vi "PathPlanner_CurrentTrigEventMarkers_FGV.vi"(10 "in EventMarkers":T1[](array[typedef]) {"lastRobotPos"."Y" format="%14.3f"; "lastRobotPos"."X" format="%14.3f"; "markerPos"."Y" format="%14.3f"; "markerPos"."X" format="%14.3f"}, 11 "Write":bool) -> (2 "out EventMarkers":T1[](array[typedef]) {"lastRobotPos"."Y" format="%14.3f"; "lastRobotPos"."X" format="%14.3f"; "markerPos"."Y" format="%14.3f"; "markerPos"."X" format="%14.3f"})   [LabVIEW 2023]
uses:
  <vilib>/Rock Robotics/WPI/ThirdParty/JAS_Junk/TrajLib/TypeDef/TRANSLATION2D.ctl
  <vilib>/Rock Robotics/WPI/ThirdParty/JAS_Junk/TrajLib/Trajectory_Library.lvlib
  <vilib>/Rock Robotics/WPI/ThirdParty/MJansen/PathPlanner/ENum/PathPlanner_CommandUtilType_ENUM.ctl
  <vilib>/Rock Robotics/WPI/ThirdParty/MJansen/PathPlanner/PathPlanner24.lvlib
  <vilib>/Rock Robotics/WPI/ThirdParty/MJansen/PathPlanner/TypeDef/PathPlannerCommandUtil.ctl
  <vilib>/Rock Robotics/WPI/ThirdParty/MJansen/PathPlanner/TypeDef/PathPlannerEventMarker.ctl
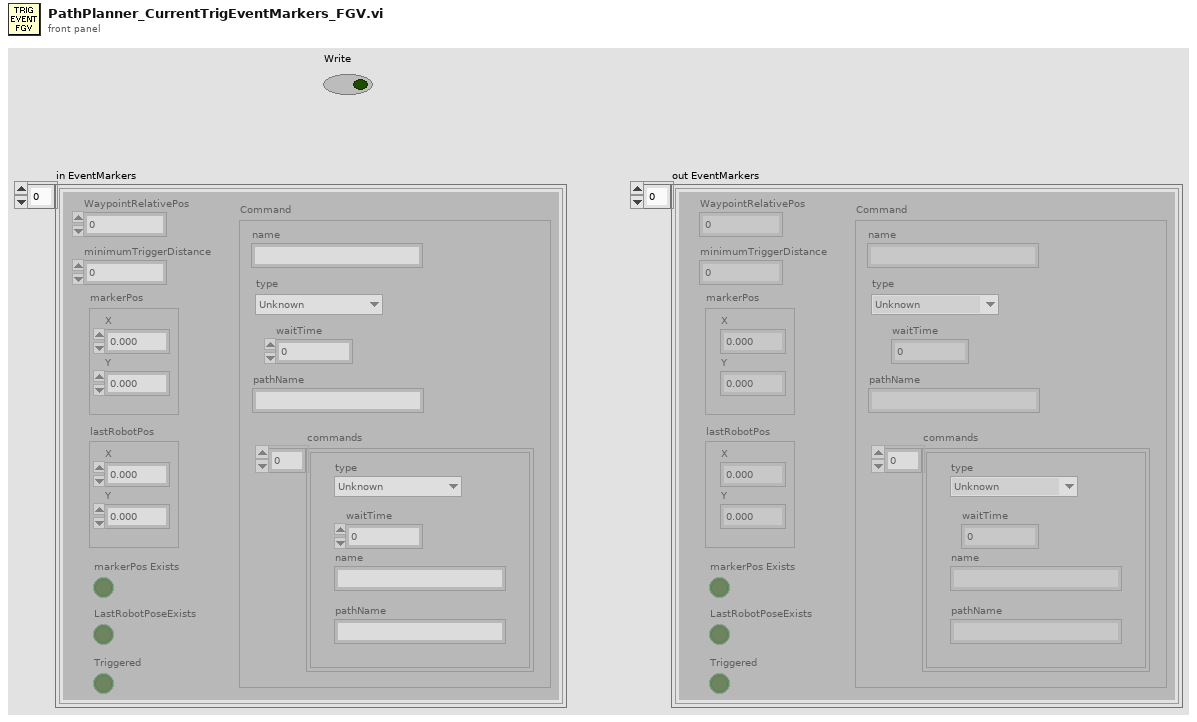
[diagram p1: front panel]
types:
  T1 = typedef "PathPlanner24.lvlib/PathPlannerEventMarker.ctl" = cluster{"WaypointRelativePos":dbl, "minimumTriggerDistance":dbl, "markerPos":T2, "lastRobotPos":T2, "Command":T3, "markerPos Exists":bool, "LastRobotPoseExists":bool, "Triggered":bool}
  T2 = typedef "Trajectory_Library.lvlib/TRANSLATION2D.ctl" = cluster{"X":dbl, "Y":dbl}
  T3 = typedef "PathPlanner24.lvlib/PathPlannerCommandUtil.ctl" = cluster{"waitTime":dbl, "name":string, "pathName":string, "commands":cluster{"type":T4, "waitTime":dbl, "name":string, "pathName":string}[], "type":T4}
  T4 = typedef "PathPlanner24.lvlib/PathPlanner_CommandUtilType_ENUM.ctl" = enum16{"Unknown", "Wait", "Named", "Path", "Sequential", "Parallel", "Race", "Deadline"}
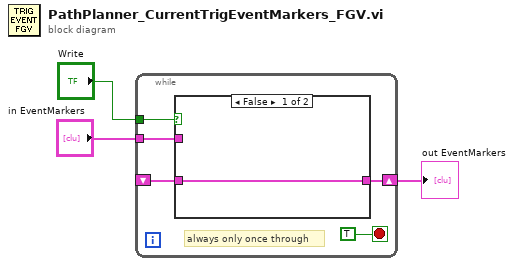
[diagram p0: block diagram]
diagram:
  n1 = while {
    tunnel: "Write" -> [w7]
    tunnel: "in EventMarkers" -> [w5]
    shift-right: [w6] -> w1
    shift-left: _ -> [w4]
    stop <- TRUE stop-if-true
    # "always only once through"
    n2 = case shown="False" w7 {
      tunnel: [w9 w10] -> w6
      tunnel: w5 -> [_ w10]
      tunnel: w4 -> [w9 _]
      frame False {
      }
      frame True {
        # "Save the trajectory\nin the shift \nregister."
      }
    }
  }
  "out EventMarkers" <- w1
